vi "ResizeTreeControltoPane.vi"(5 "Borders in Percent(T) or Pixels (F)":bool, 6 "Adjust":u16(ring) items=["Height", "Width", "Both"], 7 "Minimal":T1, 8 "error in (no error)":errorcluster, 10 "Table":refnum<vi>, 11 "Borders":T2={"Left"=116, "Top"=0, "Right"=0, "Bottom"=0}) -> (0 "error out":errorcluster)   [LabVIEW 2022 SP3, in "PentaPanesLibrary.lvlib" / "PentaPanes.lvclass"]
uses:
  PentaPanes.lvclass
  BordersCluster.ctl
  <vilib>/Utility/miscctls.llb/LVBoundsTypeDef.ctl
  <vilib>/Utility/miscctls.llb/LVPositionTypeDef.ctl
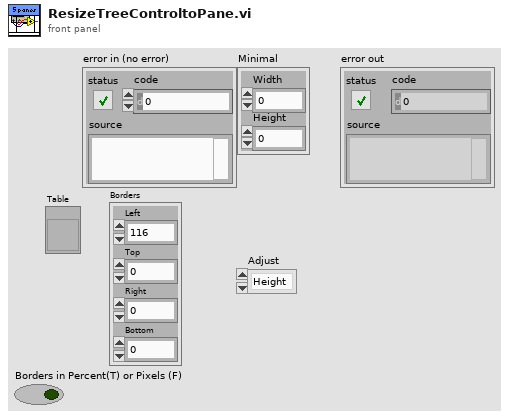
[diagram p1: front panel]
types:
  T1 = typedef "LVBoundsTypeDef.ctl" = cluster{"Width":i32, "Height":i32}
  T2 = typedef "PentaPanesLibrary.lvlib/PentaPanes.lvclass/BordersCluster.ctl" = cluster{"Left":i32, "Top":i32, "Right":i32, "Bottom":i32}
  T3 = typedef "LVPositionTypeDef.ctl" = cluster{"Left":i32, "Top":i32}
  T4 = typedef "LVBoundsTypeDef.ctl" = cluster{"Width":u32, "Height":u32}
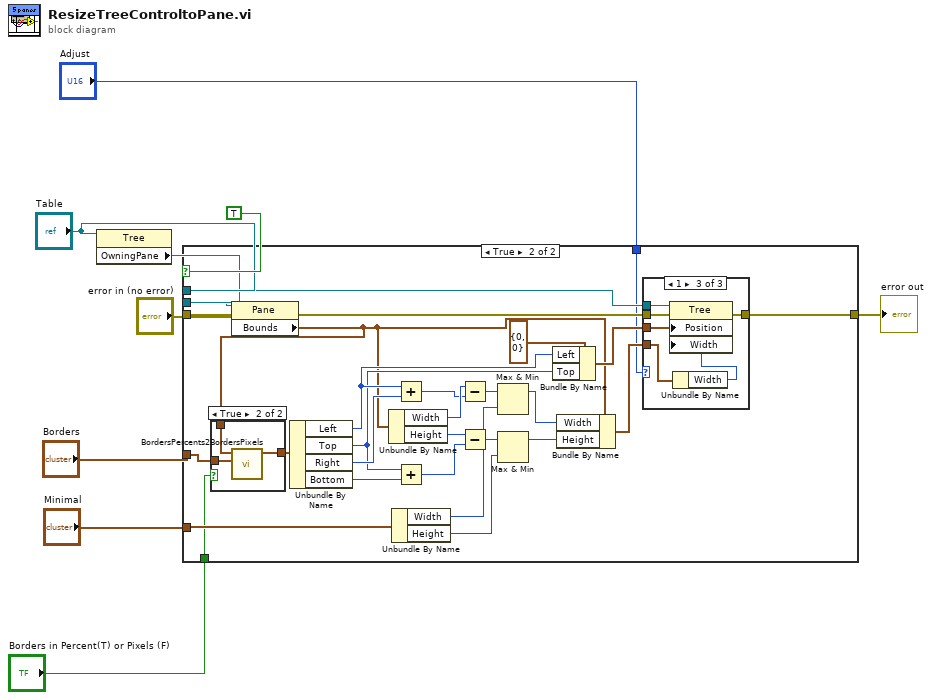
[diagram p0: block diagram]
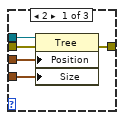
[diagram p4: hidden frame]
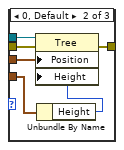
[diagram p5: hidden frame]
diagram:
  n1 = property class="Tree"(reference="Table") -> ("OwningPane"=w6:refnum<vi>)  [unwired: 1 in, 2 out]
  n2 = case shown="True" TRUE {
    tunnel: "Table" -> [_ w37]
    tunnel: w6 -> [_ w38]
    tunnel: "error in (no error)" -> [w10 w32]
    tunnel: [w10 w31] -> w8
    tunnel: "Borders" -> [_ w13]
    tunnel: "Minimal" -> [_ w14]
    tunnel: "Adjust" -> [_ w16]
    tunnel: "Borders in Percent(T) or Pixels (F)" -> [_ w11]
    frame False {
    }
    frame True {
      n3 = property class="Pane"(reference=w38, error in=w32) -> (error out=w33:errorcluster, "Bounds"=w15:T4)  [unwired: 1 out]
      n4 = case shown="True" w11 {
        tunnel: w15 -> [_ w42]
        tunnel: w13 -> [w39 w41]
        tunnel: [w39 w40] -> w12
        frame False {
        }
        frame True {
          n5 = call "BordersPercents2BordersPixels.vi"("Borders in"=w41, "Bounds"=w42) -> ("Borders out"=w40:T2)  [unwired: 9 in]
        }
      }
      n6 = Unbundle By Name(w12) -> ("Left"=w28:i32, "Top"=w23:i32, "Right"=w27:i32, "Bottom"=w22:i32)
      n7 = Unbundle By Name(w15) -> ("Width"=w26:u32, "Height"=w21:u32)
      n8 = Unbundle By Name(w14) -> ("Width"=w17:i32, "Height"=w18:i32)
      n9 = Add(x=w28, y=w27) -> (x+y=w25:i32)
      n10 = Add(x=w23, y=w22) -> (x+y=w20:i32)
      n11 = Subtract(x=w26, y=w25) -> (x-y=w24:u32)
      n12 = Subtract(x=w21, y=w20) -> (x-y=w19:u32)
      n13 = Max & Min(x=w24, y=w17) -> (max(x,y)=w36:u32)  [unwired: 1 out]
      n14 = Max & Min(x=w19, y=w18) -> (max(x,y)=w35:u32)  [unwired: 1 out]
      n15 = Bundle By Name(cluster=T3 {"Left"=0, "Top"=0} ("Position"), "Left"=w28, "Top"=w23) -> (w29:T3)
      n16 = Bundle By Name(cluster=w15, "Width"=w36, "Height"=w35) -> (w34:T4)
      n17 = case shown="1" w16 {
        tunnel: w37 -> [w47 w53 w59]
        tunnel: w34 -> [w46 w49 w55]
        tunnel: w33 -> [w45 w52 w58]
        tunnel: [w44 w51 w57] -> w31
        tunnel: w29 -> [w43 w50 w56]
        frame 2 {
          n18 = property class="Tree"(reference=w47, error in=w45, "Position"=w43, "Size"=w46) -> (error out=w44:errorcluster)  [unwired: 1 out]
        }
        frame 0, Default {
          n19 = Unbundle By Name(w49) -> ("Height"=w48:u32)
          n20 = property class="Tree"(reference=w53, error in=w52, "Position"=w50, "Height"=w48) -> (error out=w51:errorcluster)  [unwired: 1 out]
        }
        frame 1 {
          n21 = Unbundle By Name(w55) -> ("Width"=w54:u32)
          n22 = property class="Tree"(reference=w59, error in=w58, "Position"=w56, "Width"=w54) -> (error out=w57:errorcluster)  [unwired: 1 out]
        }
      }
    }
  }
  "error out" <- w8
